vi "WinCI Get Supported Capabilites.vi"(8 "error in (no error)":errorcluster) -> (0 "error out":errorcluster, 3 "suppCaps":u32)   [LabVIEW 2017, in "NI_SCC_WinCI.lvlib"]
uses:
  <vilib>/SourceControl/Providers/WinCI/NI_SCC_WinCI.lvlib
  <vilib>/SourceControl/sccapi/SCCAPI SCC Provider Functionality.ctl
  <vilib>/SourceControl/sccapi/NI_SCC.lvlib
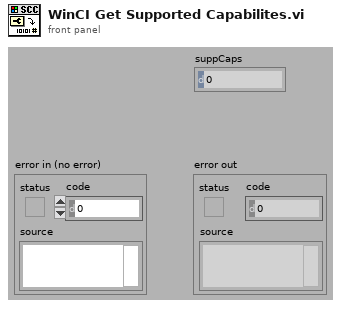
[diagram p1: front panel]
types:
  T1 = typedef "NI_SCC.lvlib/SCCAPI SCC Provider Functionality.ctl" = enum16{"Advanced - Get Latest", "Advanced - CheckOut", "Advanced - CheckIn", "Advanced - UndoCheckOut", "Advanced - Add", "Advanced - Remove", "Advanced - FileCompare", "Advanced - FileHistory", "Advanced - FileProperties", "Advanced - ConfigOptions", "Run SCC", "Configure Project", "Comment on CheckOut", "Comment on CheckIn", "Comment on Add", "Comment on Remove", "Keep Checked Out", "Get File Copy", "Multifile History"}
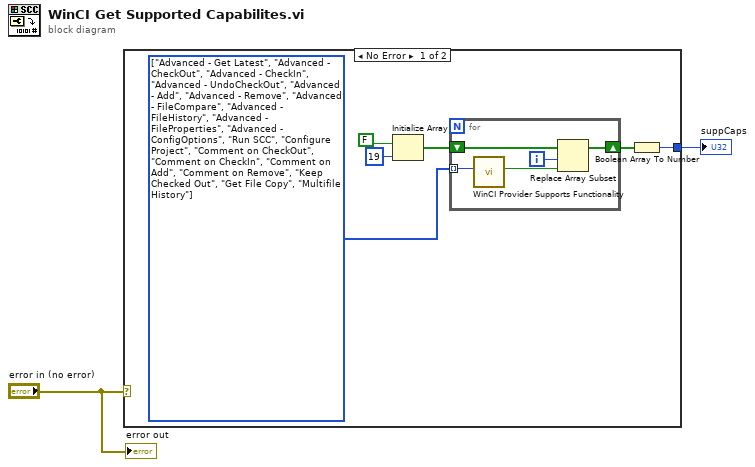
[diagram p0: block diagram]
diagram:
  n1 = case shown="No Error" "error in (no error)" {
    tunnel: [w4 _] -> w2
    frame No Error {
      w5 = T1[] [enum."Advanced - Get Latest", enum."Advanced - CheckOut", enum."Advanced - CheckIn", enum."Advanced - UndoCheckOut", enum."Advanced - Add", enum."Advanced - Remove", enum."Advanced - FileCompare", enum."Advanced - FileHistory", enum."Advanced - FileProperties", enum."Advanced - ConfigOptions", enum."Run SCC", enum."Configure Project", enum."Comment on CheckOut", enum."Comment on CheckIn", enum."Comment on Add", enum."Comment on Remove", enum."Keep Checked Out", enum."Get File Copy", enum."Multifile History"] items=["Advanced - Get Latest", "Advanced - CheckOut", "Advanced - CheckIn", "Advanced - UndoCheckOut", "Advanced - Add", "Advanced - Remove", "Advanced - FileCompare", "Advanced - FileHistory", "Advanced - FileProperties", "Advanced - ConfigOptions", "Run SCC", "Configure Project", "Comment on CheckOut", "Comment on CheckIn", "Comment on Add", "Comment on Remove", "Keep Checked Out", "Get File Copy", "Multifile History"]
      n2 = Initialize Array(FALSE, 19 ("dimension size")) -> (w6:bool[])
      n3 = for {
        shift-right: [w11] -> w3
        shift-left: w6 -> [w13]
        tunnel: w5 -> [w10] mode=indexing
        i -> [w12]
        n4 = call <vilib>:"WinCI Provider Supports Functionality.vi"("functionality"=w10) -> ("provider supports?"=w9:bool)  [unwired: 1 in, 9 out]
        n5 = Replace Array Subset(array=w13, new element=w9, index=w12) -> (w11:bool[])
      }
      n6 = Boolean Array To Number(Boolean array=w3) -> (number=w4:u32)
    }
    frame Error {
    }
  }
  "suppCaps" <- w2
  "error out" <- "error in (no error)"
